vi "change T.vi"(8 "Temperature Units (C)":u16(ring) items=["Celsius", "Fahrenheit", "Kelvin", "Rankine"], 9 "ThermocoupleType":u16(ring)=2 items=["B", "E", "J", "K", "R", "S", "T", "N"], 10 "Temperature":sgl format="%0.6f", 11 "Voltage Waveform":waveform(dbl)={"t0"=timestamp(0 s since 1904-01-01), "dt"=0.0, "Y"=[]}) -> (2 "Temperature Waveform":waveform(dbl))   [LabVIEW 2009]
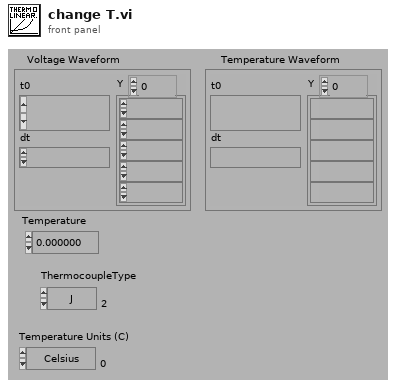
[diagram p1: front panel]
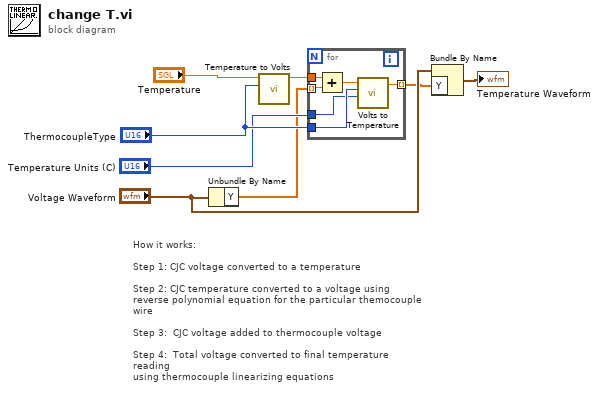
[diagram p0: block diagram]
diagram:
  # "How it works:\n\nStep 1: CJC voltage converted to a temperature\n\nStep 2: CJC temperature converted to a voltage using reverse polynomial equation for the particular themocouple wire\n\nStep 3:  CJC voltage added to thermocouple voltage\n\nStep 4:  Total voltage converted to final temperature reading \nusing thermocouple linearizing equations"
  n1 = Unbundle By Name("Voltage Waveform") -> ("Y"=w5:dbl[])
  n2 = call <vilib>:"Temperature to Volts.vi"("ThermocoupleType"="ThermocoupleType", "Temperature"="Temperature") -> ("Thermocouple Voltage"=w8:sgl)  [unwired: 1 in, 4 out]
  n3 = for {
    tunnel: [w13] -> w3 mode=indexing
    tunnel: w5 -> [w14] mode=indexing
    tunnel: w8 -> [w11]
    tunnel: "ThermocoupleType" -> [w10]
    tunnel: "Temperature Units (C)" -> [w9]
    n4 = Add(x=w11, y=w14) -> (x+y=w12:dbl)
    n5 = call <vilib>:"Volts to Temperature.vi"("Temperature Units"=w9, "ThermocoupleType"=w10, "Thermocouple Voltage"=w12) -> ("Temperature"=w13:sgl)  [unwired: 4 out]
  }
  n6 = Bundle By Name(cluster="Voltage Waveform", "Y"=w3) -> (→"Temperature Waveform":waveform(dbl))
